vi "纳清_校准命令写入.vi"(7 "探头":T1(ring), 8 "error in (no error)":errorcluster caption="错误输入（无错误）", 10 "数值":u16, 11 "MB session in":refnum<class "MB_Master.lvclass">) -> (0 "error out":errorcluster caption="错误输出", 3 "MB session out":refnum<class "MB_Master.lvclass">)   [LabVIEW 2016, in "斯坦道多参数.lvlib"]
uses:
  <vilib>/Plasmionique/MB Master/MB Master.lvlib
  <vilib>/Plasmionique/MB Master/MB_Master/MB_Master.lvclass
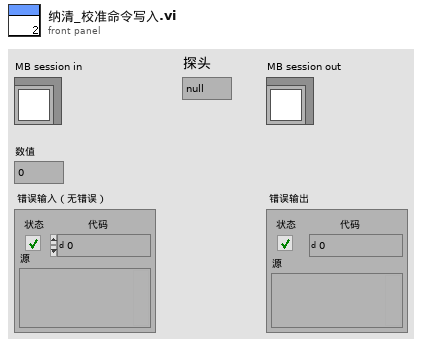
[diagram p1: front panel]
types:
  T1 = enum16{"null", "pH", "DO", "浊度", "电导率", "叶绿素a", "藻密度"}
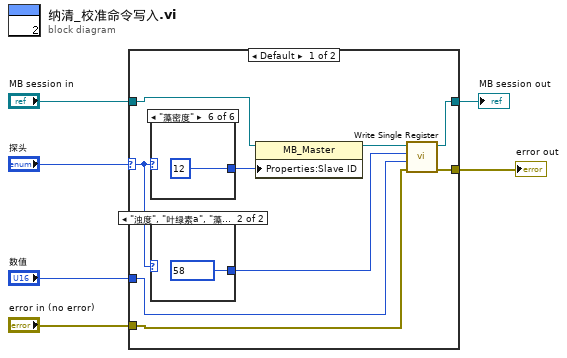
[diagram p0: block diagram]
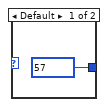
[diagram p2: hidden frame]
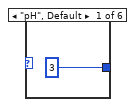
[diagram p3: hidden frame]
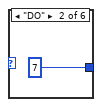
[diagram p4: hidden frame]
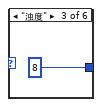
[diagram p5: hidden frame]
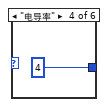
[diagram p6: hidden frame]
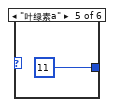
[diagram p7: hidden frame]
diagram:
  n1 = case shown="Default" "探头" {
    selector: "探头" -> [w7 _]
    tunnel: "error in (no error)" -> [w15 w24]
    tunnel: [w14 w24] -> w5
    tunnel: "数值" -> [w12 _]
    tunnel: "MB session in" -> [w11 w25]
    tunnel: [w10 w25] -> w2
    frame Default {
      n2 = case shown="\"藻密度\"" w7 {
        tunnel: [3 7 8 4 11 12] -> w9
        frame "pH", Default {
        }
        frame "DO" {
        }
        frame "浊度" {
        }
        frame "电导率" {
        }
        frame "叶绿素a" {
        }
        frame "藻密度" {
        }
      }
      n3 = case shown="\"浊度\", \"叶绿素a\", \"藻密度\"" w7 {
        tunnel: [u16 57 ("starting address") u16 58 ("starting address")] -> w8
        frame Default {
        }
        frame "浊度", "叶绿素a", "藻密度" {
        }
      }
      n4 = property class="MB_Master"(reference=w11, "Properties:Slave ID"=w9) -> (reference out=w13:refnum<class "MB_Master.lvclass">)  [unwired: 1 in, 1 out]
      n5 = call <vilib>:"Write Single Register.vi"("error in (no error)"=w15, "value"=w12, "address"=w8, "MB session in"=w13) -> ("error out"=w14:errorcluster, "MB session out"=w10:refnum<class "MB_Master.lvclass">)  [unwired: 6 in]
    }
    frame "null" {
    }
  }
  "error out" <- w5
  "MB session out" <- w2
